vi "MM6Archiver.write file.vi"(0 "i ref in":refnum<vi>, 2 "eventData":string, 5 "error in (no error)":errorcluster) -> (14 "i ref out":refnum<vi>, 19 "error out":errorcluster)   [LabVIEW 2014, in "MM6Archiver.lvlib"]
doc: "Writes one trap specific event data to a file."
uses:
  MM6Archiver.lvlib
  CS_Core/CSSystem/CoreDefs/CoreDefs.error_type.ctl
  CSData/DiscArchiver/DiscArchiver.lvlib
  CS_Core/CSSystem/CoreLib/CoreLib.lvlib
  CSlibraries/UtilityLib/UtilityLib.lvlib
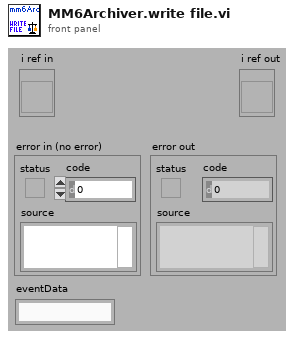
[diagram p1: front panel]
types:
  T1 = typedef "CoreDefs.error_type.ctl" = enum16{"no error", "can't load process", "can't unload process", "process does not exist", "can't install process", "can't remove process", "unknown function", "time out", "can't execute function", "duplicate queue name", "super not found", "caller queue invalid", "can't ping process", "unknown error", "VISA Error", "VISA timeout", "GPIB timeout", "GPIB error", "communication error", "data type mismatch", "can't read data from OPC server", "can't write data to OPC server", "OET error", "function not implemented", "process already exists", "invalid Shared Variable name", "error writing Shared Variable", "error reading Shared Variable", "invalid client name", "corrupt database", "unknown class", "call not authorized", "parameter out of range", "OET timeout: can't get data to modify", "invalid queue name", "requested operation incompatible with current state", "event undefined", "event disabled", "state undefined", "caller is not a friend", "EventBuilder: bad eventID", "EventBuilder: no DAQ devices", "a thread must not stop itself", "UNUSED ELEMENT4", "DiscArchiver: eventData incomplete", "DiscArchiver: eventData does not belong to run", "DiscArchiver: can't open file", "DiscArchiver: can't write to file", "DiscArchiver: available disc space low", "can't acquire semaphore", "error reading data from database", "notifier object is not existing", "can't register process", "can't unregister process", "illegal event type", "object disabled", "object already exists", "can't change state", "Instrument not found", "no connection to remote node", "invalid reference", "N/A", "UNUSED ELEMENT 1", "element not found", "illegal TCP/IP connection detected", "object does not exist", "invalid access ID", "unknown CS system", "invalid privilige", "unsupported data type", "unsupported server type", "IO server already exists", "Shared Variable already exists"}
  T2 = typedef "DiscArchiver.lvlib/DiscArchiver.i attribute.ctl" = cluster{"file prefix":string, "actual file":string, "nOfEvents":i32, "file":refnum<file>, "eventBuilder":string, "disc size alarm":bool, "dataDescription":string, "dataDescriptionURL":string, "eventDataURL":string, "headerID":dbl, "completeData":bool, "nOfEventsID":i32, "dataFileID":i32}
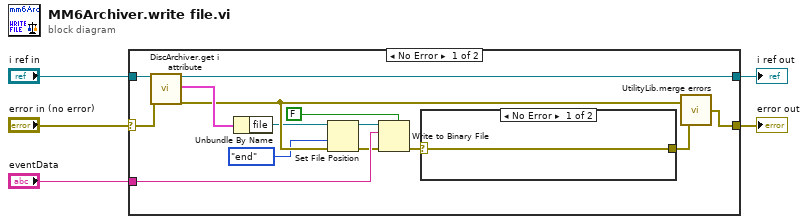
[diagram p0: block diagram]
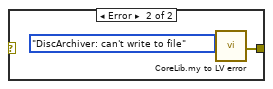
[diagram p2: hidden frame]
diagram:
  n1 = case shown="No Error" "error in (no error)" {
    selector: "error in (no error)" -> [w13 w23]
    tunnel: "i ref in" -> [w19 w24]
    tunnel: "eventData" -> [w11 _]
    tunnel: [w17 w24] -> w3
    tunnel: [w16 w23] -> w2
    frame No Error {
      n2 = call "DiscArchiver.get i attribute.vi"("i ref in"=w19, "error in (no error)"=w13) -> ("i ref out"=w17:refnum<vi>, "i attribute"=w18:T2, "error out"=w8:errorcluster)  [unwired: 15 in]
      n3 = Unbundle By Name(w18) -> ("file"=w7:refnum<file>)
      n4 = Set File Position(refnum=w7, from (0:start)=enum16{"start", "end", "current"}."end", error in=w8) -> (refnum out=w10:refnum<file>, error out=w9:errorcluster)  [unwired: 1 in]
      n5 = Write to Binary File(file (use dialog)=w10, data=w11, error in=w9, 5:FALSE ("prepend array or string size? (T)")) -> (error out=w15:errorcluster)  [unwired: 2 in, 2 out]
      n6 = case shown="No Error" w15 {
        selector: w15 -> [w20 _]
        tunnel: [w20 w22] -> w14
        frame No Error {
        }
        frame Error {
          n7 = call "CoreLib.my to LV error.vi"("ErrorTypes"=CoreDefs.error_type."DiscArchiver: can't write to file") -> ("myErrorCluster"=w22:errorcluster)  [unwired: 17 in, 1 out]
        }
      }
      n8 = call "UtilityLib.merge errors.vi"("error2 (no error)"=w14, "error1 (no error)"=w8) -> ("error out"=w16:errorcluster)
    }
    frame Error {
    }
  }
  "error out" <- w2
  "i ref out" <- w3
